vi "VI_sensor_Dashboard.vi"() -> (1 "Encoder_TracaoR":dbl, 2 "Encoder_TracaoL":dbl, 3 "NavX_Value":dbl, 4 "ElevatorEncoder":dbl, 5 "LimitSwitch":dbl)   [LabVIEW 2017]
uses:
  <vilib>/Rock Robotics/Network Tables/NT Read Number.vi
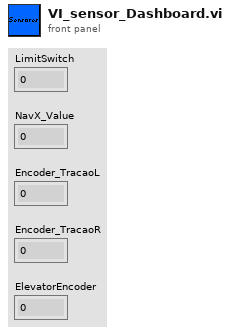
[diagram p1: front panel]
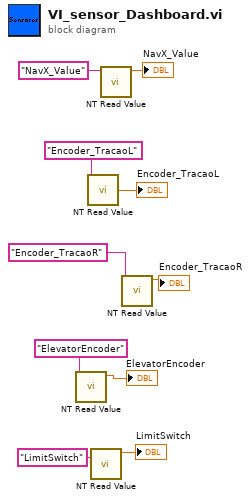
[diagram p0: block diagram]
diagram:
  n1 = call-poly <vilib>:"NT Read Value.vi"("Name"="ElevatorEncoder") -> ("Numeric"=→"ElevatorEncoder":dbl)  [unwired: 9 in, 1 out]
  n2 = call-poly <vilib>:"NT Read Value.vi"("Name"="Encoder_TracaoL") -> ("Numeric"=→"Encoder_TracaoL":dbl)  [unwired: 9 in, 1 out]
  n3 = call-poly <vilib>:"NT Read Value.vi"("Name"="LimitSwitch") -> ("Numeric"=→"LimitSwitch":dbl)  [unwired: 9 in, 1 out]
  n4 = call-poly <vilib>:"NT Read Value.vi"("Name"="NavX_Value") -> ("Numeric"=→"NavX_Value":dbl)  [unwired: 9 in, 1 out]
  n5 = call-poly <vilib>:"NT Read Value.vi"("Name"="Encoder_TracaoR") -> ("Numeric"=→"Encoder_TracaoR":dbl)  [unwired: 9 in, 1 out]
